vi "Reset checkpoint.vi"(8 "error in (no error)":errorcluster, 11 "Autofocus in":refnum<class "Autofocus.lvclass">) -> (0 "error out":errorcluster, 3 "Autofocus out":refnum<class "Autofocus.lvclass">)   [LabVIEW 2012, in "Autofocus.lvclass"]
uses:
  Autofocus.lvclass
  Autofocus.lvclass/Autofocus.ctl
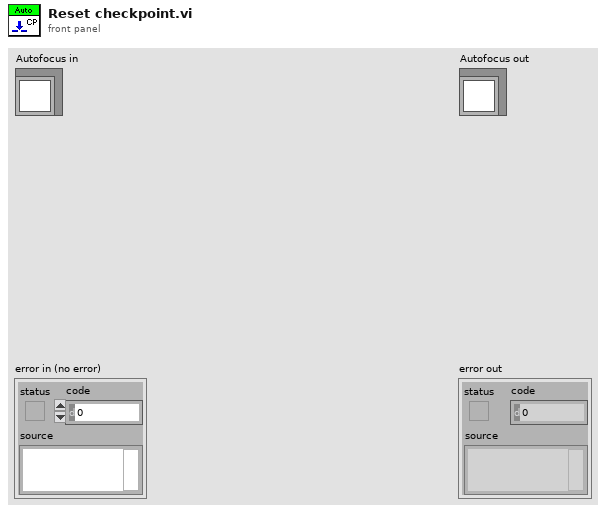
[diagram p1: front panel]
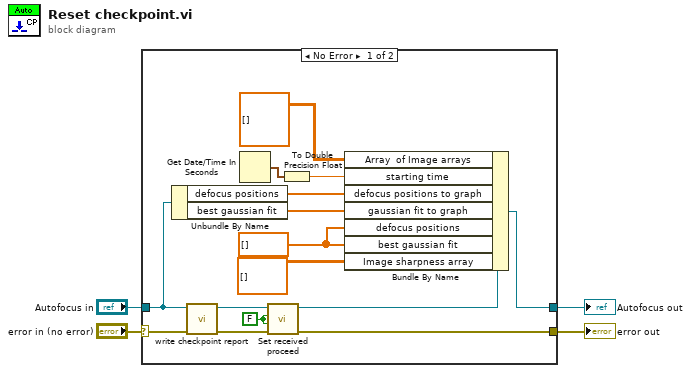
[diagram p0: block diagram]
diagram:
  n1 = case shown="No Error" "error in (no error)" {
    selector: "error in (no error)" -> [w14 w21]
    tunnel: [w18 w21] -> w3
    tunnel: [w16 w20] -> w1
    tunnel: "Autofocus in" -> [w12 w20]
    frame No Error {
      w6 = dbl[] [] ("Runtime cluster.Checkpoint .Image sharpness array")
      w19 = FALSE ("from stage?")
      n2 = Unbundle By Name(w12) -> ("defocus positions"=w15:dbl[], "best gaussian fit"=w5:dbl[])
      n3 = call-dynamic "write checkpoint report.vi"("error in (no error)"=w14, "Autofocus in"=w12) -> ("error out"=w13:errorcluster, "Autofocus out"=w11:refnum<class "Autofocus.lvclass">)  [unwired: 8 in]
      n4 = Get Date/Time In Seconds() -> (seconds since 1Jan1904=w10:timestamp)
      n5 = call-dynamic "Set received proceed.vi"("error in (no error)"=w13, "from camera?"=w19, "from stage?"=w19, "Autofocus in"=w11) -> ("error out"=w18:errorcluster, "Autofocus out"=w17:refnum<class "Autofocus.lvclass">)  [unwired: 6 in]
      n6 = To Double Precision Float(number=w10) -> (double precision float=w9:dbl)
      n7 = Bundle By Name(cluster=w17, "Array  of Image arrays"=dbl[][][] [] ("Runtime cluster.Image.Array  of Image arrays"), "starting time"=w9, "defocus positions to graph"=w15, "gaussian fit to graph"=w5, "defocus positions"=w6, "best gaussian fit"=w6, "Image sharpness array"=dbl[][] [] ("Runtime cluster.Checkpoint .Image sharpness array")) -> (w16:refnum<class "Autofocus.lvclass">)
    }
    frame Error {
    }
  }
  "error out" <- w3
  "Autofocus out" <- w1
